vi "CRYSet Search Ranges.vi"(10 "Search Items":string[](array[string]), 11 "Type":enum16{"Curves", "Values", "Results", "WFM"}(ring)) -> (0 "Checks":bool[](array[boolean]), 1 "Caption":string, 2 "Item Names":string[](array[string]), 3 "Symbols":i32[](array[numeric]))   [LabVIEW 2013]
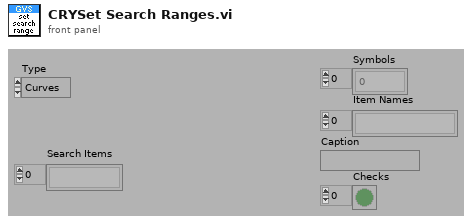
[diagram p1: front panel]
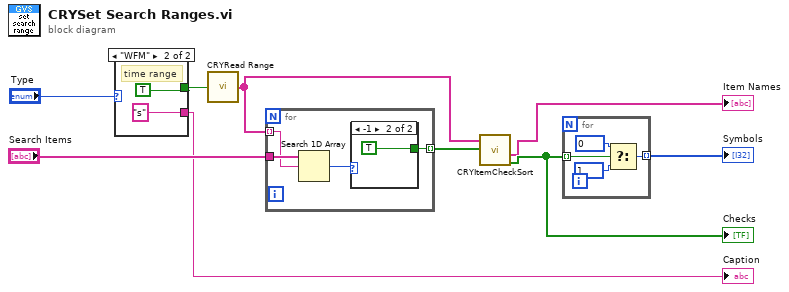
[diagram p0: block diagram]
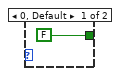
[diagram p2: hidden frame]
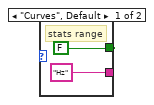
[diagram p3: hidden frame]
diagram:
  n1 = case shown="\"WFM\"" "Type" {
    tunnel: ["Hz" ("Caption.Text") "s" ("Caption.Text")] -> w5
    tunnel: [FALSE ("In s<->Hz") TRUE ("In s<->Hz")] -> w7
    frame "Curves", Default {
      # "stats range"
    }
    frame "WFM" {
      # "time range"
    }
  }
  "Caption" <- w5
  n2 = call "CRYRead Range.vi"("In s<->Hz"=w7) -> ("Out Search_Range"=w4:string[])
  n3 = for {
    tunnel: w4 -> [w14] mode=indexing
    tunnel: [w17] -> w3 mode=indexing
    tunnel: "Search Items" -> [w15]
    n4 = Search 1D Array(1D array=w15, element=w14) -> (index of element=w16:i32)  [unwired: 1 out]
    n5 = case shown="-1" w16 {
      tunnel: [FALSE TRUE] -> w17
      frame 0, Default {
      }
      frame -1 {
      }
    }
  }
  n6 = call "CRYItemCheckSort.vi"("Check_s"=w3, "In Items"=w4) -> ("Out Check"=w2:bool[], "Out Items"=→"Item Names":string[])  [unwired: 6 in, 2 out]
  "Checks" <- w2
  n7 = for {
    tunnel: w2 -> [w23] mode=indexing
    tunnel: [w22] -> w9 mode=indexing
    n8 = Select(t=0, s=w23, f=1) -> (s? t:f=w22:i32)
  }
  "Symbols" <- w9
